vi "Save Data.vi"(7 "Folder to save file to":path=path "C:/Users/LAV-UFSC-2023/Documents/LAV-TCC/Dados-Experimentos/Dados-Bancada-LABVIEW", 8 "error in (no error)":errorcluster, 11 "Data":waveform(dbl)[](array[waveform])) -> (0 "error out":errorcluster)   [LabVIEW 2022 SP3]
doc: "Saves data to disk."
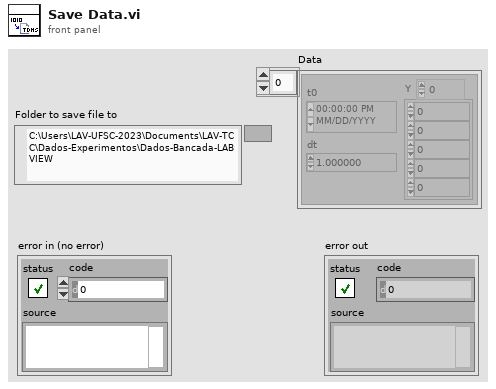
[diagram p1: front panel]
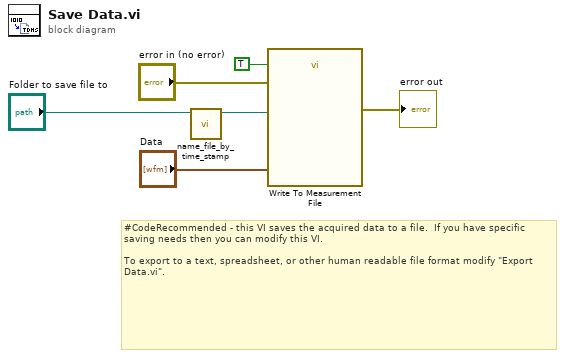
[diagram p0: block diagram]
diagram:
  # "#CodeRecommended - this VI saves the acquired data to a file.  If you have specific saving needs then you can modify this VI.\n\nTo export to a text, spreadsheet, or other human readable file format modify \"Export Data.vi\"."
  n1 = call "name_file_by_time_stamp.vi"("Folder to save file to"="Folder to save file to") -> ("New file path"=w2:path)  [unwired: 10 in]
  n2 = call "Write To Measurement File"("Signals"="Data", "Reset"=TRUE, "error in (no error)"="error in (no error)", "Filename"=w2) -> ("error out"=→"error out":errorcluster)  [unwired: 13 in, 2 out]
